vi "ReadNmeaData.vi"(8 "error in":errorcluster, 9 "Airmar Wind Queue Cluster":T2, 10 "GPS-Compass Queue Cluster":T3, 11 "Serial Port":refnum<visa-resource-name>) -> (0 "error out":errorcluster, 1 "Read string":string, 2 "GPS DATA VALID?":bool, 3 "Robot UTM Location":T1 {"North" format="%#_10f"; "East" format="%#_8f"}, 4 "GPS STRING":string[](array[string]), 5 "Boat Direction 2":dbl, 7 "Relative Wind Direction":dbl)   [LabVIEW 2013]
uses:
  Data/TypeDefs/GPS-Compass Queue Cluster.ctl
  Data/TypeDefs/UTM Location.ctl
  Data/TypeDefs/WindData Queue Cluster.ctl
panel:
  out "Pitch 2":dbl
  out "Roll 2":dbl
  out "Pitch":dbl
  out "Roll":dbl
  out "Wind Speed (m/s)":dbl
  out "Absolute Wind Direction":dbl
  out "Rate Of Turn (deg/s)":dbl
  out "Boat Direction":dbl
  out "Boat Velocity Direction":dbl
  out "Boat Speed":dbl
  out "Longitude":dbl
  out "Latitude":dbl
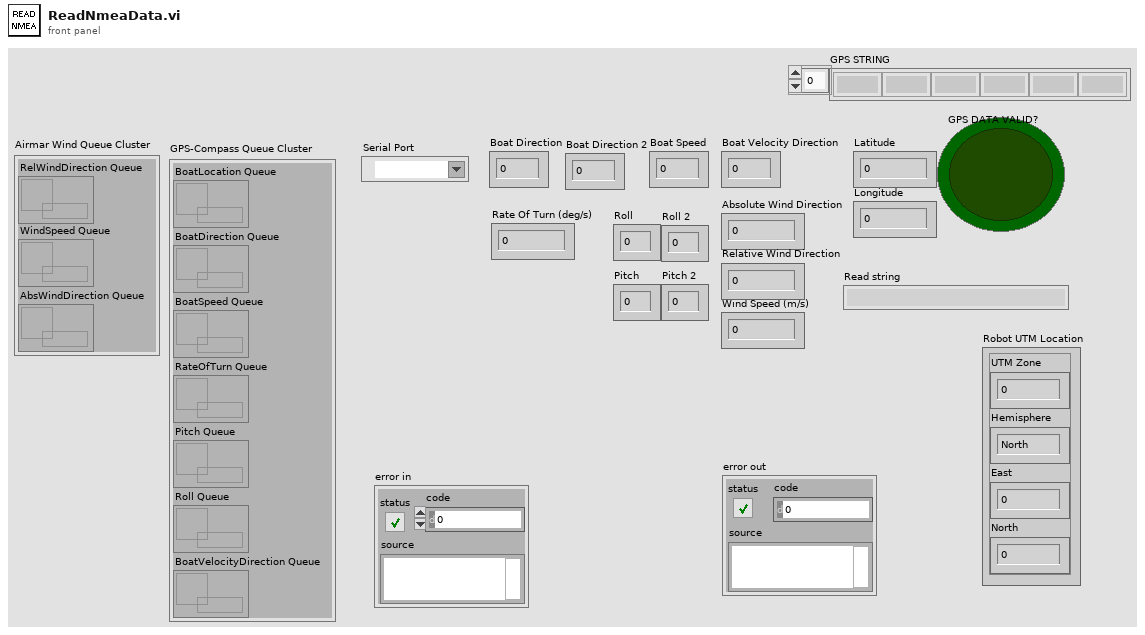
[diagram p1: front panel]
types:
  T1 = typedef "UTM Location.ctl" = cluster{"UTM Zone":dbl, "Hemisphere":enum16{"North", "South"}, "East":dbl, "North":dbl}
  T2 = typedef "WindData Queue Cluster.ctl" = cluster{"RelWindDirection Queue":refnum<queue>, "WindSpeed Queue":refnum<queue>, "AbsWindDirection Queue":refnum<queue>}
  T3 = typedef "GPS-Compass Queue Cluster.ctl" = cluster{"BoatLocation Queue":refnum<queue>, "BoatDirection Queue":refnum<queue>, "BoatSpeed Queue":refnum<queue>, "RateOfTurn Queue":refnum<queue>, "Pitch Queue":refnum<queue>, "Roll Queue":refnum<queue>, "BoatVelocityDirection Queue ":refnum<queue>}
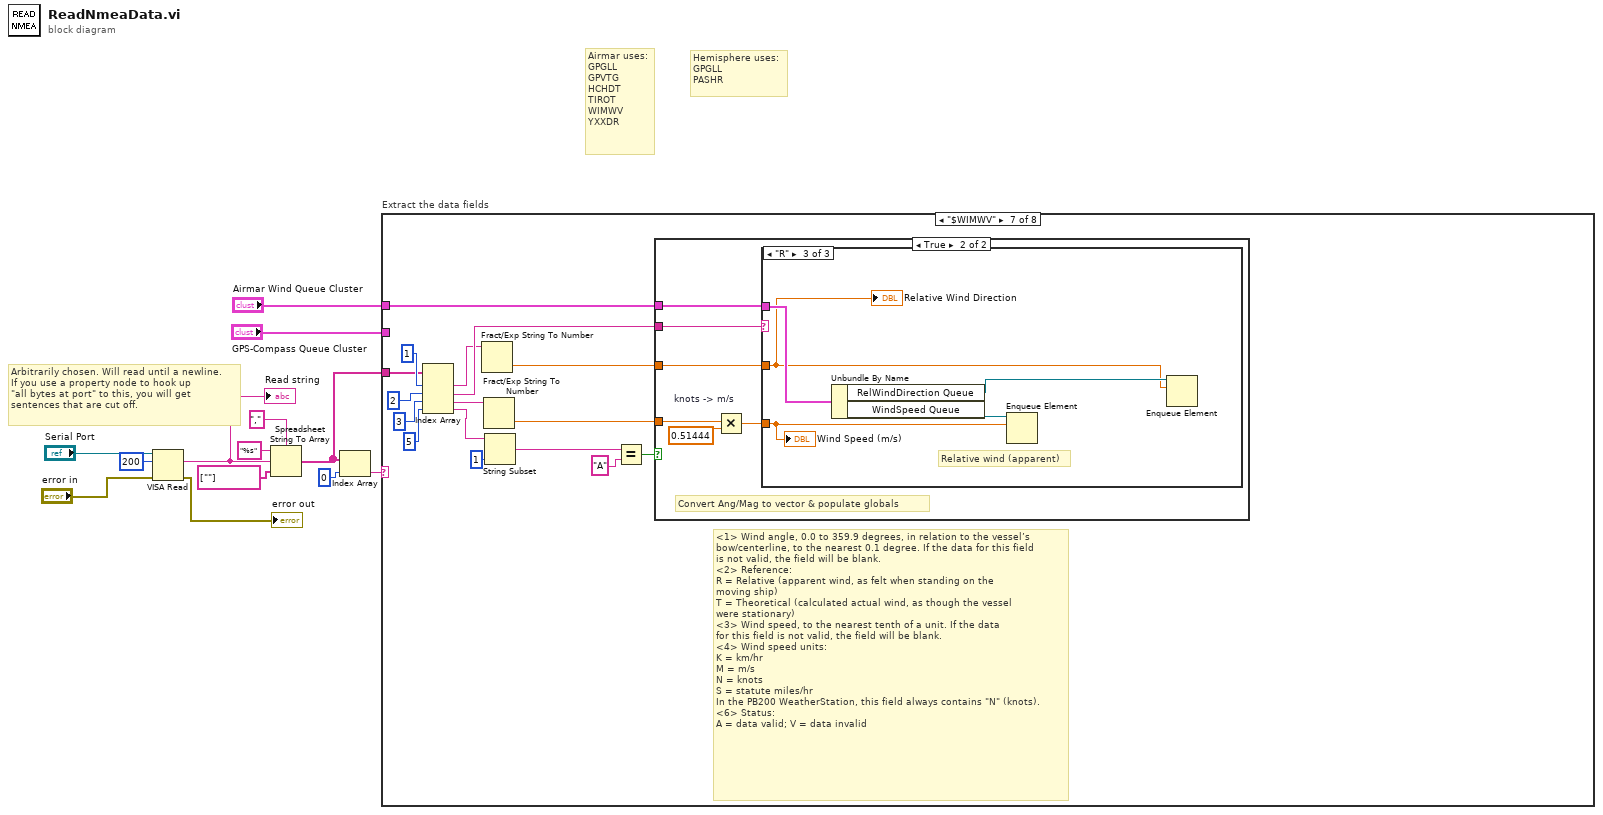
[diagram p0: block diagram]
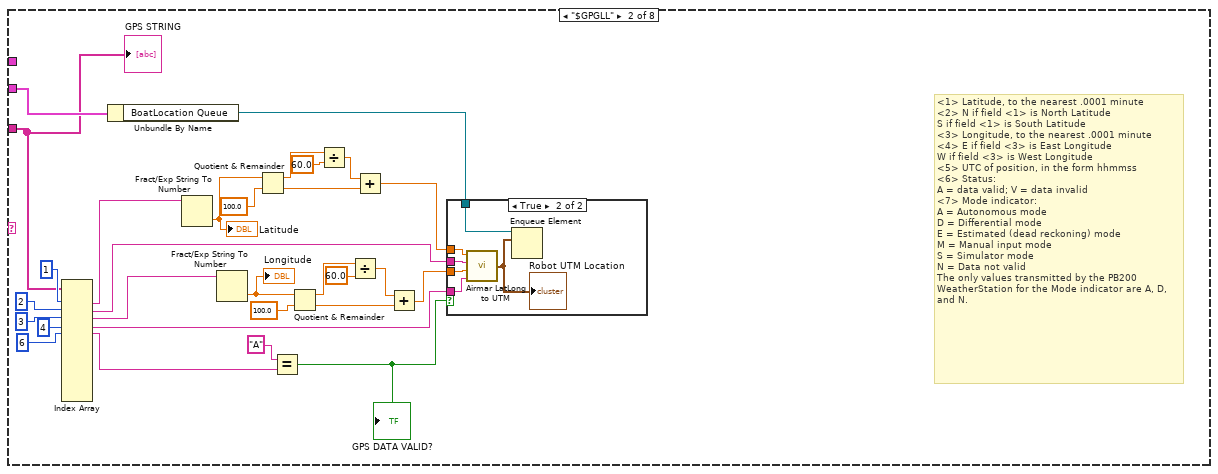
[diagram p3: hidden frame]
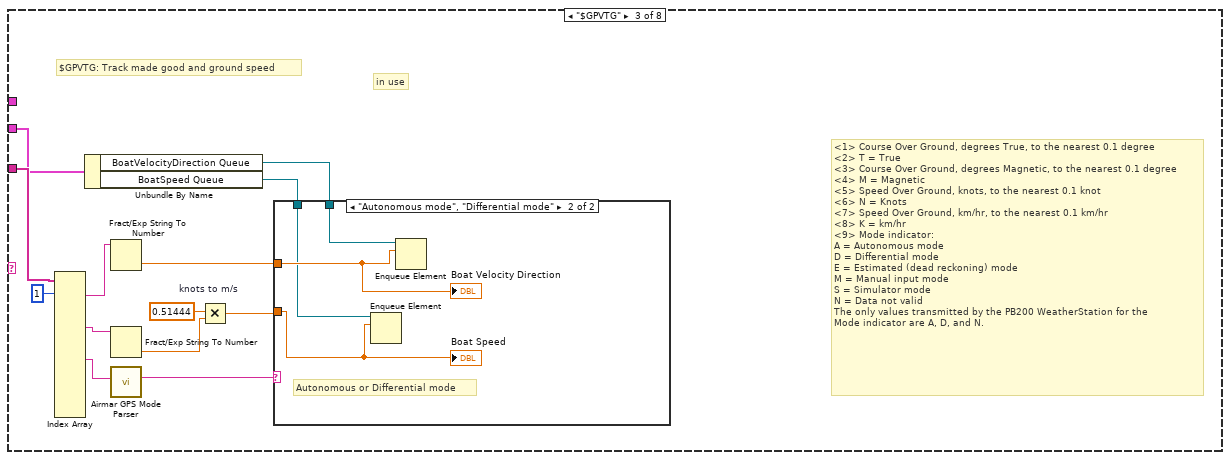
[diagram p5: hidden frame]
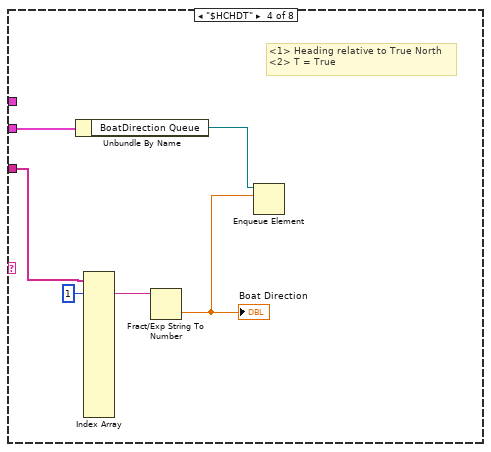
[diagram p7: hidden frame]
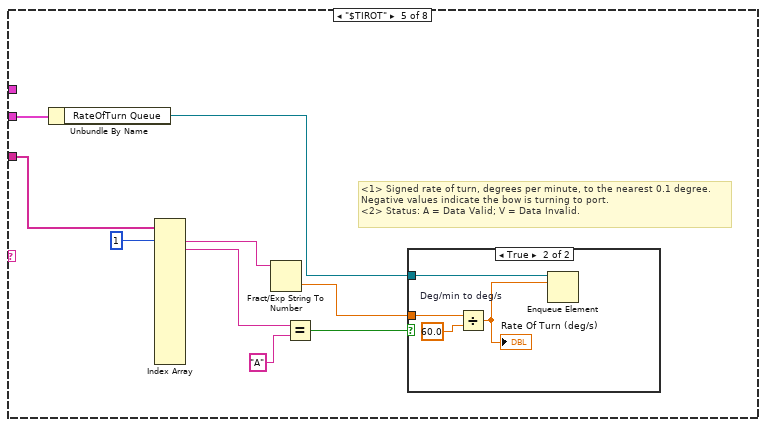
[diagram p8: hidden frame]
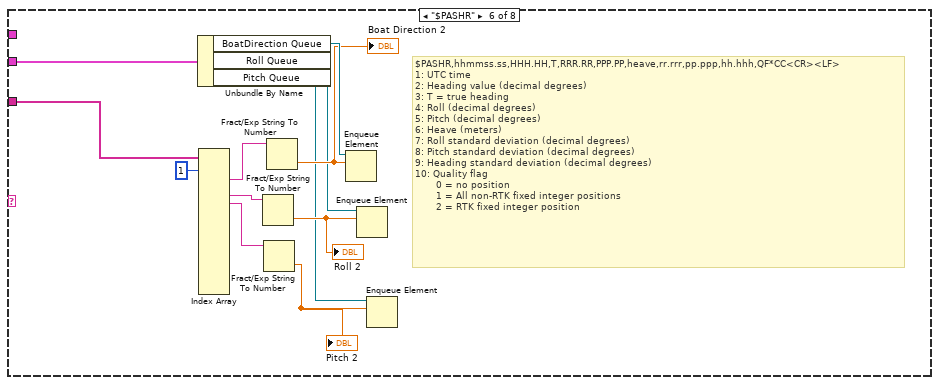
[diagram p10: hidden frame]
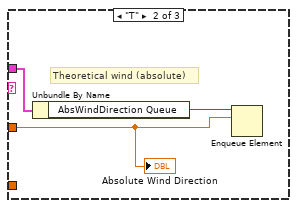
[diagram p13: hidden frame]
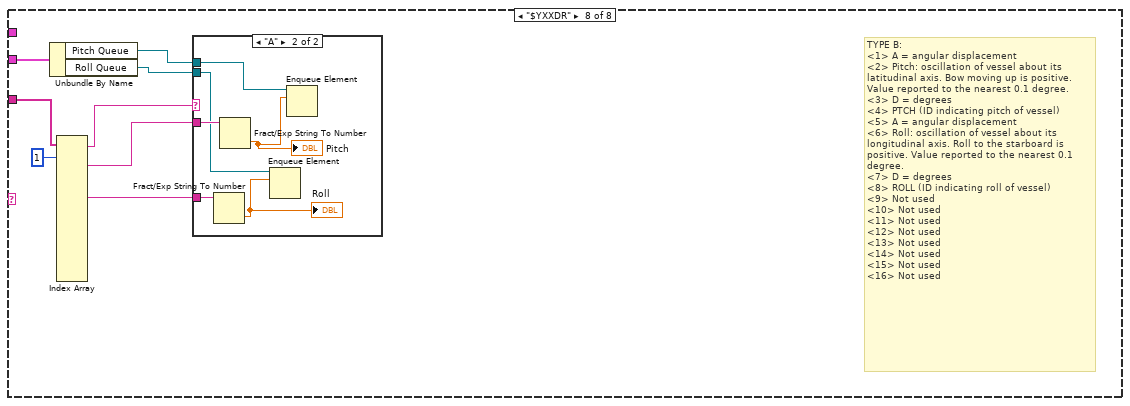
[diagram p14: hidden frame]
diagram:
  # "Hemisphere uses:\nGPGLL\nPASHR"
  # "Airmar uses:\nGPGLL\nGPVTG\nHCHDT\nTIROT\nWIMWV\nYXXDR"
  # "Arbitrarily chosen. Will read until a newline.\nIf you use a property node to hook up\n\"all bytes at port\" to this, you will get \nsentences that are cut off."
  n1 = VISA Read(VISA resource name="Serial Port", byte count=u32 200, error in (no error)="error in") -> (read buffer=w2:string, error out=→"error out":errorcluster)  [unwired: 2 out]
  "Read string" <- w2
  n2 = Spreadsheet String To Array(delimiter (Tab)=",", format string="%s", spreadsheet string=w2, array type (2D Dbl)=string[] [""]) -> (array=w1:string[])
  n3 = Index Array(array=w1, index=0) -> (element=w6:string)
  n4 = case "Extract the data fields" shown="\"$WIMWV\"" w6 {
    tunnel: w1 -> [_ w14 w61 w71 w78 w85 w105 w134]
    tunnel: "GPS-Compass Queue Cluster" -> [_ w22 w51 w68 w73 w86 _ w129]
    tunnel: "Airmar Wind Queue Cluster" -> [_ _ _ _ _ _ w106 _]
    frame Default {
      # "Unknown sentence."
    }
    frame "$GPGLL" {
      # "<1> Latitude, to the nearest .0001 minute\n<2> N if field <1> is North Latitude\nS if field <1> is South Latitude\n<3> Longitude, to the nearest .0001 minute\n<4> E if field <3> is East Longitude\nW if field <3> is West Longitude\n<5> UTC of position, in the form hhmmss\n<6> Status:\nA = data valid; V = data invalid\n<7> Mode indicator:\nA = Autonomous mode\nD = Differential mode\nE = Estimated (dead reckoning) mode\nM = Manual input mode\nS = Simulator mode\nN = Data not valid\nThe only values transmitted by the PB200 WeatherStation for the Mode indicator are A, D, and N."
      n5 = Index Array(array=w14, index #1=1 ("index"), index #2=2 ("index"), index #3=3 ("index"), index #4=4 ("index"), index #5=6 ("index")) -> (element #1=w41:string, element #2=w20:string, element #3=w40:string, element #4=w39:string, element #5=w19:string)  [unwired: 8 in, 8 out]
      n6 = Unbundle By Name(w22) -> ("BoatLocation Queue"=w21:refnum<queue>)
      n7 = Fract/Exp String To Number(string=w41) -> (number=w31:dbl)  [unwired: 3 in, 1 out]
      "Latitude" <- w31
      n8 = Fract/Exp String To Number(string=w40) -> (number=w24:dbl)  [unwired: 3 in, 1 out]
      "Longitude" <- w24
      n9 = Quotient & Remainder(x=w31, y=100.0) -> (x-y*floor(x/y)=w35:dbl, floor(x/y)=w32:dbl)
      n10 = Equal?(x="A" ("y"), y=w19) -> (x = y?=w37:bool)
      "GPS DATA VALID?" <- w37
      n11 = Quotient & Remainder(x=w24, y=100.0) -> (x-y*floor(x/y)=w28:dbl, floor(x/y)=w26:dbl)
      n12 = Divide(x=w35, y=60.0) -> (x/y=w33:dbl)
      n13 = Divide(x=w28, y=60.0) -> (x/y=w27:dbl)
      n14 = Add(x=w33, y=w32) -> (x+y=w30:dbl)
      n15 = Add(x=w27, y=w26) -> (x+y=w25:dbl)
      n16 = case shown="True" w37 {
        tunnel: w20 -> [_ w48]
        tunnel: w25 -> [_ w47]
        tunnel: w39 -> [_ w46]
        tunnel: w30 -> [_ w45]
        tunnel: w21 -> [_ w44]
        frame False {
        }
        frame True {
          n17 = call "Airmar LatLong to UTM.vi"("East/West"=w46, "Longitude"=w47, "North/South"=w48, "Latitude"=w45) -> ("Robot UTM Location"=w43:T1)
          "Robot UTM Location" <- w43
          n18 = Enqueue Element(queue=w44, element=w43) -> ()  [unwired: 2 in, 3 out]
        }
      }
      "GPS STRING" <- w14
    }
    frame "$GPVTG" {
      # "<1> Course Over Ground, degrees True, to the nearest 0.1 degree\n<2> T = True\n<3> Course Over Ground, degrees Magnetic, to the nearest 0.1 degree\n<4> M = Magnetic\n<5> Speed Over Ground, knots, to the nearest 0.1 knot\n<6> N = Knots\n<7> Speed Over Ground, km/hr, to the nearest 0.1 km/hr\n<8> K = km/hr\n<9> Mode indicator:\nA = Autonomous mode\nD = Differential mode\nE = Estimated (dead reckoning) mode\nM = Manual input mode\nS = Simulator mode\nN = Data not valid\nThe only values transmitted by the PB200 WeatherStation for the\nMode indicator are A, D, and N."
      # "in use"
      # "$GPVTG: Track made good and ground speed"
      n19 = Index Array(array=w61, index #1=1 ("index")) -> (element #1=w59:string, element #5=w58:string, element #9=w57:string)  [unwired: 15 in, 13 out]
      n20 = Unbundle By Name(w51) -> ("BoatVelocityDirection Queue"=w50:refnum<queue>, "BoatSpeed Queue"=w49:refnum<queue>)
      n21 = Fract/Exp String To Number(string=w59) -> (number=w56:dbl)  [unwired: 3 in, 1 out]
      n22 = Fract/Exp String To Number(string=w58) -> (number=w54:dbl)  [unwired: 3 in, 1 out]
      n23 = call "Airmar GPS Mode Parser.vi"("GPS Mode (Char)"=w57) -> ("GPS Mode (Description)"=w52:string)  [unwired: 6 in]
      n24 = Multiply "knots to m/s"(x=0.51444 ("y"), y=w54) -> (x*y=w55:dbl)
      n25 = case shown="\"Autonomous mode\", \"Differential mode\"" w52 {
        tunnel: w56 -> [_ w64]
        tunnel: w55 -> [_ w63]
        tunnel: w50 -> [_ w65]
        tunnel: w49 -> [_ w62]
        frame "Data not valid", Default {
          # "Data not valid"
        }
        frame "Autonomous mode", "Differential mode" {
          # "Autonomous or Differential mode"
          n26 = Enqueue Element(queue=w62, element=w63) -> ()  [unwired: 2 in, 3 out]
          n27 = Enqueue Element(queue=w65, element=w64) -> ()  [unwired: 2 in, 3 out]
          "Boat Velocity Direction" <- w64
          "Boat Speed" <- w63
        }
      }
    }
    frame "$HCHDT" {
      # "<1> Heading relative to True North\n<2> T = True"
      n28 = Unbundle By Name(w68) -> ("BoatDirection Queue"=w67:refnum<queue>)
      n29 = Index Array(array=w71, index #1=1 ("index")) -> (element #1=w70:string)  [unwired: 15 in, 15 out]
      n30 = Fract/Exp String To Number(string=w70) -> (number=w66:dbl)  [unwired: 3 in, 1 out]
      "Boat Direction" <- w66
      n31 = Enqueue Element(queue=w67, element=w66) -> ()  [unwired: 2 in, 3 out]
    }
    frame "$TIROT" {
      # "<1> Signed rate of turn, degrees per minute, to the nearest 0.1 degree.\nNegative values indicate the bow is turning to port.\n<2> Status: A = Data Valid; V = Data Invalid."
      n32 = Unbundle By Name(w73) -> ("RateOfTurn Queue"=w72:refnum<queue>)
      n33 = Index Array(array=w78, index #1=1 ("index")) -> (element #1=w77:string, element #2=w75:string)  [unwired: 15 in, 14 out]
      n34 = Fract/Exp String To Number(string=w77) -> (number=w79:dbl)  [unwired: 3 in, 1 out]
      n35 = Equal?(x=w75, y="A") -> (x = y?=w80:bool)
      n36 = case shown="True" w80 {
        tunnel: w79 -> [_ w84]
        tunnel: w72 -> [_ w81]
        frame False {
        }
        frame True {
          n37 = Divide "Deg/min to deg/s"(x=w84, y=60.0) -> (x/y=w82:dbl)
          "Rate Of Turn (deg/s)" <- w82
          n38 = Enqueue Element(queue=w81, element=w82) -> ()  [unwired: 2 in, 3 out]
        }
      }
    }
    frame "$PASHR" {
      # "$PASHR,hhmmss.ss,HHH.HH,T,RRR.RR,PPP.PP,heave,rr.rrr,pp.ppp,hh.hhh,QF*CC<CR><LF>\n1: UTC time\n2: Heading value (decimal degrees)\n3: T = true heading\n4: Roll (decimal degrees)\n5: Pitch (decimal degrees)\n6: Heave (meters)\n7: Roll standard deviation (decimal degrees)\n8: Pitch standard deviation (decimal degrees)\n9: Heading standard deviation (decimal degrees)\n10: Quality flag\n       0 = no position\n       1 = All non-RTK fixed integer positions\n       2 = RTK fixed integer position"
      n39 = Unbundle By Name(w86) -> ("BoatDirection Queue"=w95:refnum<queue>, "Roll Queue"=w91:refnum<queue>, "Pitch Queue"=w90:refnum<queue>)
      n40 = Index Array(array=w85, index #1=1 ("index")) -> (element #2=w94:string, element #4=w89:string, element #5=w88:string)  [unwired: 15 in, 13 out]
      n41 = Fract/Exp String To Number(string=w89) -> (number=w92:dbl)  [unwired: 3 in, 1 out]
      "Roll 2" <- w92
      n42 = Fract/Exp String To Number(string=w88) -> (number=w87:dbl)  [unwired: 3 in, 1 out]
      "Pitch 2" <- w87
      n43 = Fract/Exp String To Number(string=w94) -> (number=w93:dbl)  [unwired: 3 in, 1 out]
      "Boat Direction 2" <- w93
      n44 = Enqueue Element(queue=w95, element=w93) -> ()  [unwired: 2 in, 3 out]
      n45 = Enqueue Element(queue=w91, element=w92) -> ()  [unwired: 2 in, 3 out]
      n46 = Enqueue Element(queue=w90, element=w87) -> ()  [unwired: 2 in, 3 out]
    }
    frame "$WIMWV" {
      # "<1> Wind angle, 0.0 to 359.9 degrees, in relation to the vessel’s\nbow/centerline, to the nearest 0.1 degree. If the data for this field\nis not valid, the field will be blank.\n<2> Reference:\nR = Relative (apparent wind, as felt when standing on the\nmoving ship)\nT = Theoretical (calculated actual wind, as though the vessel\nwere stationary)\n<3> Wind speed, to the nearest tenth of a unit. If the data\nfor this field is not valid, the field will be blank.\n<4> Wind speed units:\nK = km/hr\nM = m/s\nN = knots\nS = statute miles/hr\nIn the PB200 WeatherStation, this field always contains \"N\" (knots).\n<6> Status:\nA = data valid; V = data invalid"
      n47 = Index Array(array=w105, index #1=1 ("index"), index #2=2 ("index"), index #3=3 ("index"), index #4=5 ("index")) -> (element #1=w97:string, element #2=w104:string, element #3=w111:string, element #4=w98:string)
      n48 = Fract/Exp String To Number(string=w97) -> (number=w110:dbl)  [unwired: 3 in, 1 out]
      n49 = Fract/Exp String To Number(string=w111) -> (number=w109:dbl)  [unwired: 3 in, 1 out]
      n50 = String Subset(string=w98, length (rest)=1 ("length (rest)")) -> (substring=w102:string)  [unwired: 1 in]
      n51 = Equal?(x=w102, y="A") -> (x = y?=w108:bool)
      n52 = case shown="True" w108 {
        tunnel: w109 -> [_ w115]
        tunnel: w110 -> [_ w118]
        tunnel: w104 -> [_ w117]
        tunnel: w106 -> [_ w113]
        frame False {
        }
        frame True {
          # "Convert Ang/Mag to vector & populate globals"
          n53 = Multiply "knots -> m/s"(x=w115, y=0.51444) -> (x*y=w116:dbl)
          n54 = case shown="\"R\"" w117 {
            tunnel: w116 -> [_ _ w124]
            tunnel: w118 -> [_ w119 w122]
            tunnel: w113 -> [_ w121 w126]
            frame "", Default {
            }
            frame "T" {
              # "Theoretical wind (absolute)"
              n55 = Unbundle By Name(w121) -> ("AbsWindDirection Queue"=w120:refnum<queue>)
              n56 = Enqueue Element(queue=w120, element=w119) -> ()  [unwired: 2 in, 3 out]
              "Absolute Wind Direction" <- w119
            }
            frame "R" {
              # "Relative wind (apparent)"
              n57 = Unbundle By Name(w126) -> ("RelWindDirection Queue"=w123:refnum<queue>, "WindSpeed Queue"=w125:refnum<queue>)
              n58 = Enqueue Element(queue=w125, element=w124) -> ()  [unwired: 2 in, 3 out]
              n59 = Enqueue Element(queue=w123, element=w122) -> ()  [unwired: 2 in, 3 out]
              "Relative Wind Direction" <- w122
              "Wind Speed (m/s)" <- w124
            }
          }
        }
      }
    }
    frame "$YXXDR" {
      # "TYPE B:\n<1> A = angular displacement\n<2> Pitch: oscillation of vessel about its latitudinal axis. Bow moving up is positive. Value reported to the nearest 0.1 degree.\n<3> D = degrees\n<4> PTCH (ID indicating pitch of vessel)\n<5> A = angular displacement\n<6> Roll: oscillation of vessel about its longitudinal axis. Roll to the starboard is positive. Value reported to the nearest 0.1 degree.\n<7> D = degrees\n<8> ROLL (ID indicating roll of vessel)\n<9> Not used\n<10> Not used\n<11> Not used\n<12> Not used\n<13> Not used\n<14> Not used\n<15> Not used\n<16> Not used"
      n60 = Unbundle By Name(w129) -> ("Pitch Queue"=w128:refnum<queue>, "Roll Queue"=w127:refnum<queue>)
      n61 = Index Array(array=w134, index #1=1 ("index")) -> (element #1=w133:string, element #2=w131:string, element #6=w130:string)  [unwired: 15 in, 13 out]
      n62 = case shown="\"A\"" w133 {
        tunnel: w131 -> [_ w140]
        tunnel: w130 -> [_ w139]
        tunnel: w128 -> [_ w138]
        tunnel: w127 -> [_ w136]
        frame "", Default {
        }
        frame "A" {
          n63 = Fract/Exp String To Number(string=w139) -> (number=w135:dbl)  [unwired: 3 in, 1 out]
          "Roll" <- w135
          n64 = Fract/Exp String To Number(string=w140) -> (number=w137:dbl)  [unwired: 3 in, 1 out]
          "Pitch" <- w137
          n65 = Enqueue Element(queue=w136, element=w135) -> ()  [unwired: 2 in, 3 out]
          n66 = Enqueue Element(queue=w138, element=w137) -> ()  [unwired: 2 in, 3 out]
        }
      }
    }
  }
